vi "Process Monitor.vi"(0 "Index":i32=100) -> (1 "Pressure":dbl=0.03536048750581487 format="%.2f", 2 "Temperature":dbl=79.58984375 format="%.2f", 3 "Volume":dbl=80.15776548385574 format="%.2f")   [LabVIEW 2022 SP3]
panel:
  in  "Simulated Temp Data":i32[](array[numeric])=[163, 163, 163, 163, 163, 163, 165, 169, 172, 173, 172, 172, 171, 171, 174, 176, 177, 178, 178, 179, 178, 177, 176, 175, 175, 174, 173, 172, 172, 172, 172, 172, 171, 171, 170, 170, 170, 172, 173, 174, 175, 177, 178, 178, 178, 177, 176, 175, 176, 178, 179, 180, 179, 178, 178, 176, 176, 176, 174, 174, 174, 173, 173, 175, 176, 178, 178, 177, 176, 175, 175, 174, 174, 173, 173, 172, 172, 171, 171, 170, 170, 170, 170, 170, 170, 170, 169, 166, 167, 169, 170, 169, 168, 168, 168, 168, 167, 167, 167, 167]
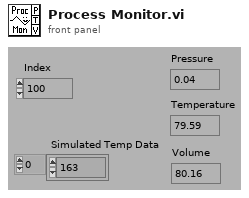
[diagram p1: front panel]
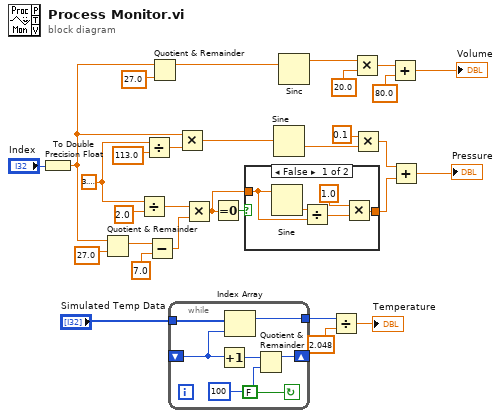
[diagram p0: block diagram]
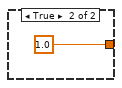
[diagram p2: hidden frame]
diagram:
  w18 = 3.141592653589793
  n1 = To Double Precision Float(number="Index") -> (double precision float=w6:dbl)
  n2 = Quotient & Remainder(x=w6, y=27.0) -> (x-y*floor(x/y)=w21:dbl)  [unwired: 1 out]
  n3 = Divide(x=w18, y=2.0) -> (x/y=w23:dbl)
  n4 = Divide(x=w18, y=113.0) -> (x/y=w27:dbl)
  n5 = Subtract(x=w21, y=7.0) -> (x-y=w24:dbl)
  n6 = Quotient & Remainder(x=w6, y=27.0) -> (x-y*floor(x/y)=w13:dbl)  [unwired: 1 out]
  n7 = while {
    tunnel: "Simulated Temp Data" -> [w32]
    tunnel: [w33] -> w4
    shift-left: _ -> [w37]
    shift-right: [w34] -> _
    stop <- FALSE continue-if-true
    n8 = Increment(x=w37) -> (x+1=w36:i32)
    n9 = Index Array(array=w32, index=w37) -> (element=w33:i32)
    n10 = Quotient & Remainder(x=w36, y=100) -> (x-y*floor(x/y)=w34:i32)  [unwired: 1 out]
  }
  n11 = Multiply(x=w6, y=w27) -> (x*y=w16:dbl)
  n12 = Multiply(x=w23, y=w24) -> (x*y=w26:dbl)
  n13 = Equal To 0?(x=w26) -> (x = 0?=w25:bool)
  n14 = case shown="False" w25 {
    tunnel: [w40 1.0] -> w15
    tunnel: w26 -> [w41 _]
    frame False {
      n15 = Sine(x=w41) -> (sin(x)=w42:dbl)
      n16 = Divide(x=w42, y=w41) -> (x/y=w38:dbl)
      n17 = Multiply(x=1.0, y=w38) -> (x*y=w40:dbl)
    }
    frame True {
    }
  }
  n18 = Sine(x=w16) -> (sin(x)=w28:dbl)
  n19 = Sinc(1:w13) -> (0:w12:dbl)
  n20 = Divide(x=w4, y=2.048) -> (x/y=→"Temperature":dbl)
  n21 = Multiply(x=w12, y=20.0) -> (x*y=w10:dbl)
  n22 = Multiply(x=0.1, y=w28) -> (x*y=w17:dbl)
  n23 = Add(x=w10, y=80.0) -> (x+y=→"Volume":dbl)
  n24 = Add(x=w17, y=w15) -> (x+y=→"Pressure":dbl)
